vi "TEST_Timer.vi"() -> ()   [LabVIEW 2024]
panel:
  out "Timed Out":bool
  out "TO Trigger":bool
  in  "Auto Reset":bool=TRUE
  in  "Reset":bool
  out "Running":bool
  out "Lap (sec)":dbl
  out "Eleapse Time (sec)":dbl
  in  "Time (sec)":dbl=3.0
  in  "Start":bool
  in  "stop":bool
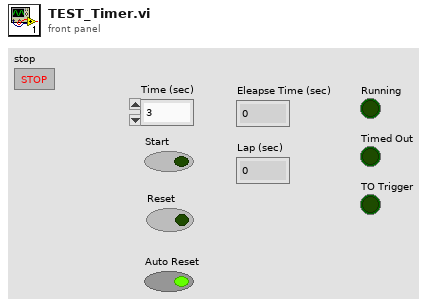
[diagram p1: front panel]
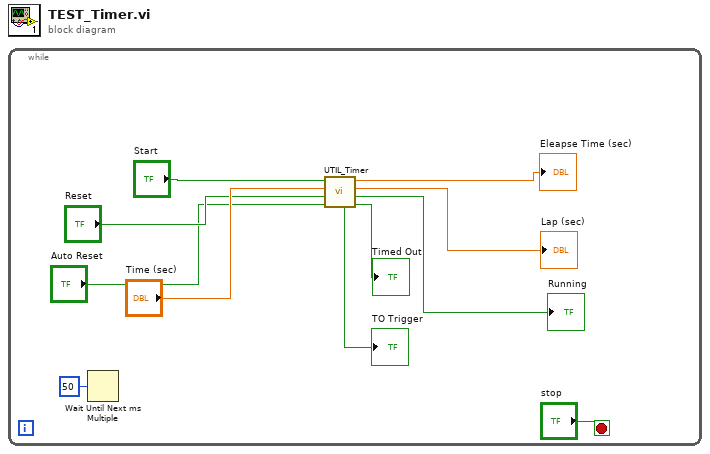
[diagram p0: block diagram]
diagram:
  n1 = while {
    stop <- "stop" stop-if-true
    n2 = Wait Until Next ms Multiple(millisecond multiple=u32 50) -> ()  [unwired: 1 out]
    n3 = call "UTIL_Timer.vi"("Auto Reset"="Auto Reset", "Reset"="Reset", "Time (sec)"="Time (sec)", "Start"="Start") -> ("Timed Out"=→"Timed Out":bool, "Running"=→"Running":bool, "Numeric 2"=→"Lap (sec)":dbl, "Numeric"=→"Eleapse Time (sec)":dbl, "TO Trig"=→"TO Trigger":bool)  [unwired: 3 in]
  }
